vi "Create Test Configuration.vi"() -> (0 "error out":errorcluster, 1 "Names":string[](array[string]), 2 "Line Array":T1[](array[typedef]), 3 "Module Configuration":refnum<class "UI Reference configuration.lvclass">, 4 "Channels":refnum<class "TBM channel.lvclass">[](array[class]), 5 "instance identifier":string)   [LabVIEW 2014, in "UI Reference tests.lvlib"]
doc: "This VI creates a standard test configuration for other unit tests. It currently creates and adds one line with every datatype to the module configuration."
uses:
  UI Reference tests.lvlib
  module/configuration/UI Reference configuration.lvclass
  <vilib>/NI/Configuration Framework/serializable configuration/NISE_CEF_serializable configuration.lvclass
  <vilib>/NI/Tag Bus Module Framework/channel/TBM channel.lvclass
  module/configuration/Line.ctl
  Test UI.vi
  <vilib>/NI/Tag Bus/tag/tag descriptor.lvclass
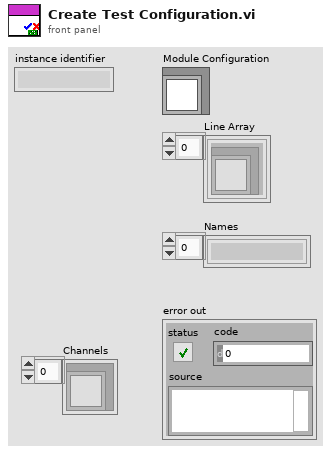
[diagram p1: front panel]
types:
  T1 = typedef "UI Reference configuration.lvclass/Line.ctl" = cluster{"channel":refnum<class "TBM channel.lvclass">}
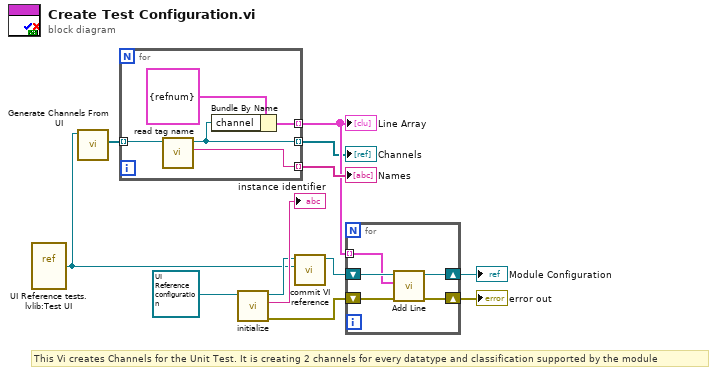
[diagram p0: block diagram]
diagram:
  # "This Vi creates Channels for the Unit Test. It is creating 2 channels for every datatype and classification supported by the module"
  n1 = vi-ref "UI Reference tests.lvlib:Test UI.vi"() -> (w2:refnum<vi>)
  n2 = call "Generate Channels From UI.vi"("VI Refnum"=w2) -> ("channels"=w1:refnum<class "TBM channel.lvclass">[])  [unwired: 9 in, 1 out]
  n3 = for {
    tunnel: [w13] -> w5 mode=indexing
    tunnel: [w15] -> w7 mode=indexing
    tunnel: [w16] -> w6 mode=indexing
    tunnel: w1 -> [w14] mode=indexing
    n4 = call <vilib>:"read tag name.vi"("system tag in"=w14) -> ("name"=w15:string, "system tag out"=w13:refnum<class "TBM channel.lvclass">)  [unwired: 8 in, 1 out]
    n5 = Bundle By Name(cluster=T1 {"channel"=refnum} ("Line"), "channel"=w13) -> (w16:T1)
  }
  "Names" <- w7
  "Line Array" <- w6
  "Channels" <- w5
  n6 = call <vilib>:"initialize.vi"("configuration in"=refnum<class "UI Reference configuration.lvclass"> refnum ("tag bus configurable plugin module configuration")) -> ("error out"=w10:errorcluster, "identifier"=→"instance identifier":string, "configuration out"=w4:refnum<class "UI Reference configuration.lvclass">)  [unwired: 8 in]
  n7 = call "commit VI reference.vi"("VI Refnum in"=w2, "UI Reference configuration in"=w4) -> ("UI Reference configuration out"=w3:refnum<class "UI Reference configuration.lvclass">)  [unwired: 7 in, 2 out]
  n8 = for {
    tunnel: w6 -> [w18] mode=indexing
    shift-right: [w21] -> w9
    shift-left: w3 -> [w22]
    shift-right: [w19] -> w12
    shift-left: w10 -> [w20]
    n9 = call "Add Line.vi"("error in"=w20, "Line"=w18, "UI Reference configuration in"=w22) -> ("error out"=w19:errorcluster, "UI Reference configuration out"=w21:refnum<class "UI Reference configuration.lvclass">)  [unwired: 6 in, 1 out]
  }
  "error out" <- w12
  "Module Configuration" <- w9
